vi "从数组中删除相同的数据.vi"(8 "带删除的相同元素在二维数组中所在的列":i32, 10 "元素":string, 11 "数组":string[][](array[string])) -> (0 "找到的元素个数":i32, 3 "输出数组":string[][](array[string]))   [LabVIEW 2017]
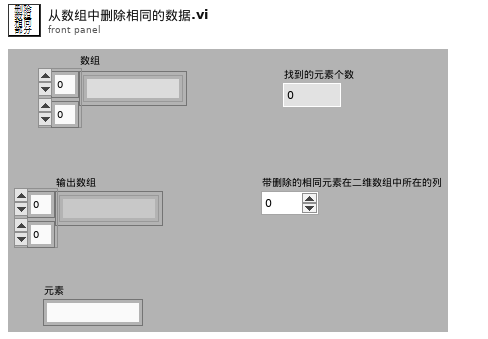
[diagram p1: front panel]
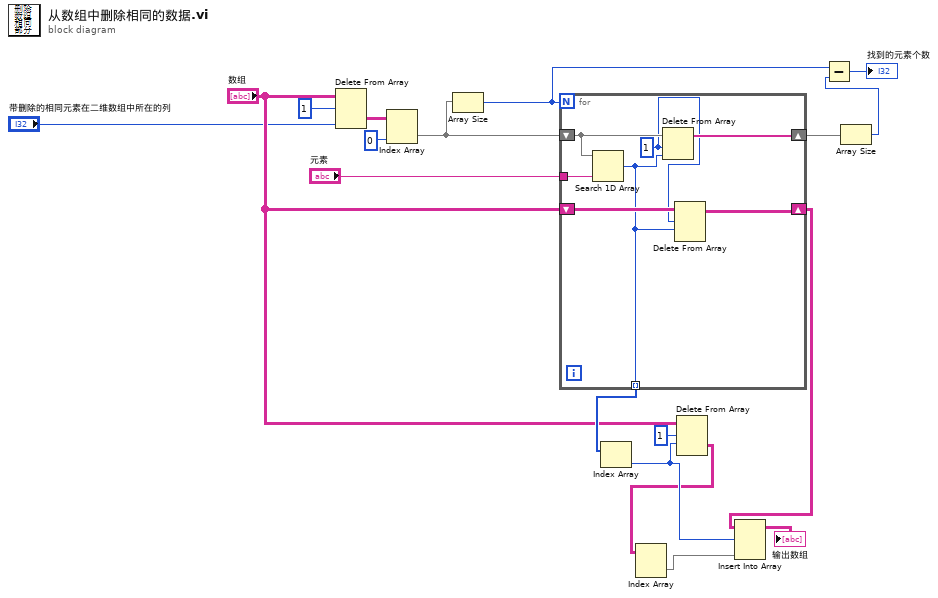
[diagram p0: block diagram]
diagram:
  n1 = Delete From Array(array="数组", length=1 ("长度"), index (col)="带删除的相同元素在二维数组中所在的列") -> (deleted portion=w17:string[][])  [unwired: 1 in, 1 out]
  n2 = Index Array(array=w17, index (col)=0 ("索引 (行)")) -> (element=w16:string[])  [unwired: 1 in]
  n3 = Array Size(array=w16) -> (size(s)=w10:i32)
  n4 = for {
    N: w10 -> [_]
    tunnel: "元素" -> [w25]
    shift-right: [w24] -> w11
    shift-left: w16 -> [w23]
    shift-right: [w22] -> w2
    shift-left: "数组" -> [w21]
    tunnel: [w19] -> w8 mode=indexing
    w20 = 1 ("长度")
    n5 = Search 1D Array(1D array=w23, element=w25) -> (index of element=w19:i32)  [unwired: 1 in]
    n6 = Delete From Array(array=w23, length=w20, index=w19) -> (array with subset deleted=w24:string[])  [unwired: 1 out]
    n7 = Delete From Array(array=w21, length=w20, index (row)=w19) -> (array with subset deleted=w22:string[][])  [unwired: 1 in, 1 out]
  }
  n8 = Index Array(array=w8) -> (element=w6:i32)  [unwired: 1 in]
  n9 = Delete From Array(array="数组", length=1 ("长度"), index (row)=w6) -> (deleted portion=w5:string[][])  [unwired: 1 in, 1 out]
  n10 = Index Array(array=w5) -> (element=w4:string[])  [unwired: 2 in]
  n11 = Insert Into Array(array=w2, index (row)=w6, new element=w4) -> (→"输出数组":string[][])  [unwired: 1 in]
  n12 = Array Size(array=w11) -> (size(s)=w14:i32)
  n13 = Subtract(x=w10, y=w14) -> (x-y=→"找到的元素个数":i32)
